vi "Project-1.vi"() -> ()   [LabVIEW 2017]
uses:
  <vilib>/Utility/miscctls.llb/LVPositionTypeDef.ctl
  Control 2.ctl
  System.Speech
panel:
  out "?":bool
  out "?":bool
  out "?":bool
  out "?":bool
  out "Nagasandra":bool
  out "?":bool
  out "?":bool
  out "?":bool
  out "?":bool
  out "Peenya":bool
  out "?":bool
  out "Yeshwantpur":bool
  out "?":bool
  out "Nadaprabhu\nKemepowda, Majestic":bool
  out "National \nCollege":bool
  out "?":bool
  out "?":bool
  out "Jayanagar":bool
  out "?":bool
  out "?":bool
  out "?":bool
  out "?":bool
  out "?":bool
  out "?":bool
  out "Rashtriya Vidyalaya Road":bool
  out "?":bool
  out "Banashankari":bool
  out "?":bool
  out "Jaya Prakash Nagar":bool
  out "TRAIN":bool
  in  "Stop":bool
  out "Yelachenahalli":bool
  # "Yelachenahalli"
  # "Jaya Prakash Nagar"
  # "Banashankari"
  # "Rashtriya Vidyalaya Road"
  # "Jayanagar"
  # "National College"
  # "Nadaprabhu Kempegowda \n     Station, Majestic"
  # "Yeshwantpur"
  # "Peenya"
  # "Nagasandra"
  # "Rashtriya Vidyalaya Road"
  # "Jaya Prakash Nagar"
  # "National College"
  # "Nagasandra"
  # "Yeshwantpur"
  # "Dockyard"
  # "Yelachenahalli"
  # "Nadaprabhu Kempegowda \n     Station, Majestic"
  # "Banashankari"
  # "Jayanagar"
  # "Peenya"
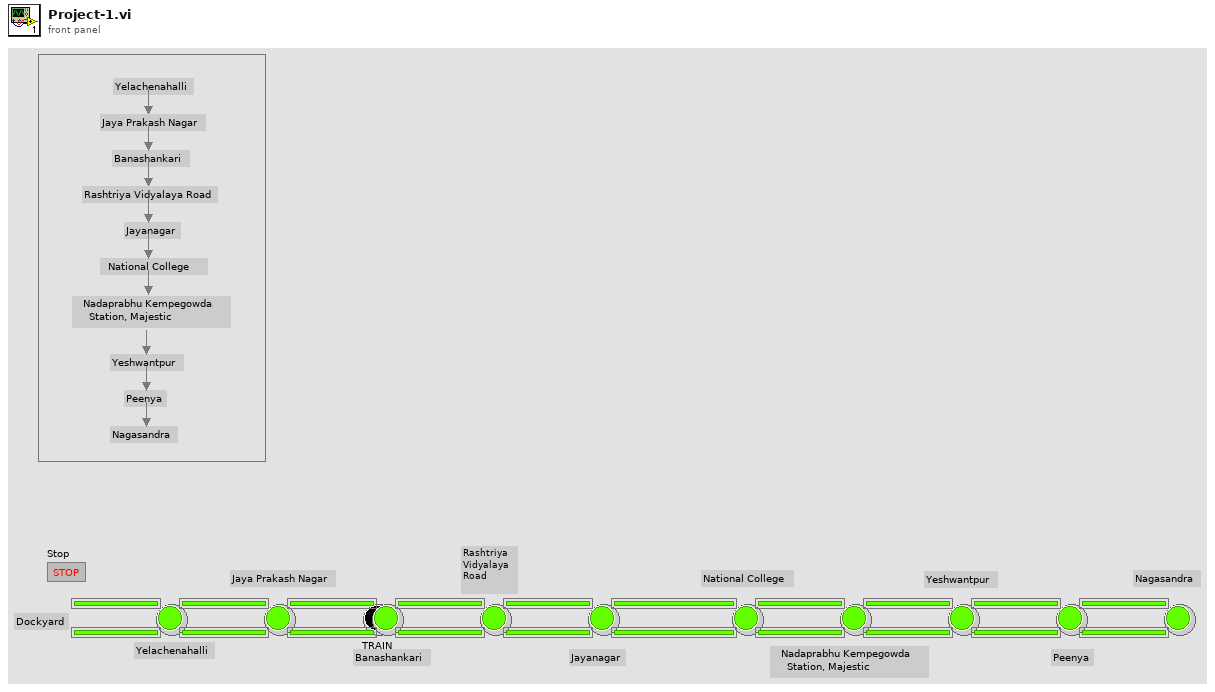
[diagram p1: front panel]
types:
  T1 = typedef "Control 2.ctl" = enum16{"Yelachenahalli", "Jaya Prakash Nagar", "Banashankari", "Rashtriya Vidyalaya Road", "Jayanagar", "National College", "Nadaprabhu Kempegowda Station. Majestic", "Yeshwantpur", "Peenya", "Nagasandra", "Return to Peenya", "Return to Yeshwantpur", "Return to Nadaprabhu Kempegowda Station, Majestic", "Return to National College", "Return to Jayanagar", "Return to Rashtriya Vidyalaya Road", "Return to Banashankari", "Return to Jaya Prakash Nagar", "Return to Yelachenahalli ", "Stop"}
  T2 = typedef "LVPositionTypeDef.ctl" = cluster{"Left":i32, "Top":i32}
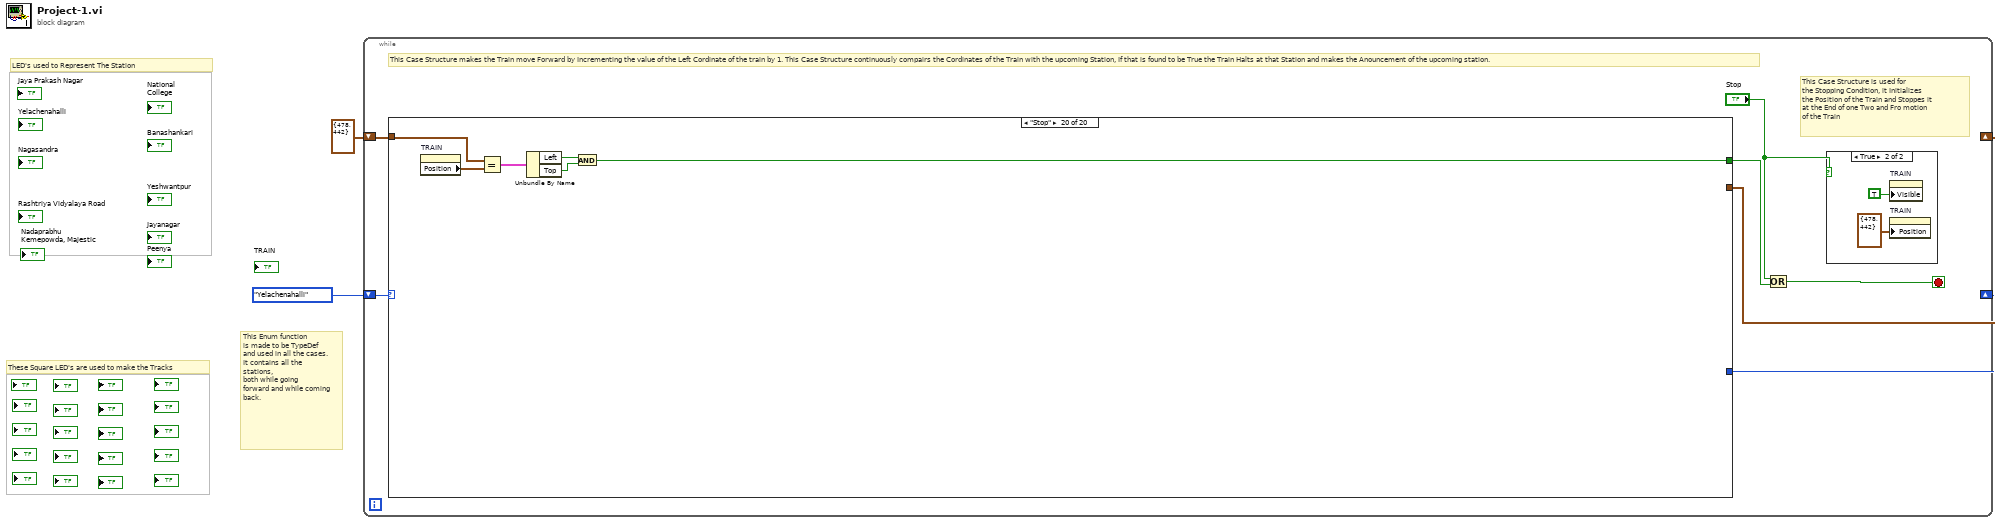
[diagram p0: block diagram]
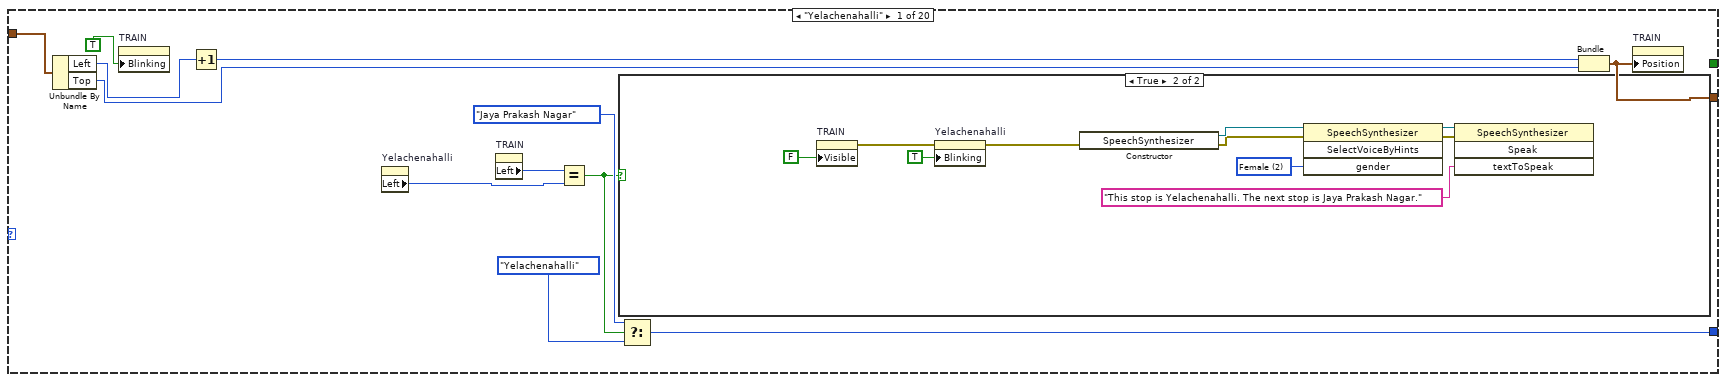
[diagram p2: hidden frame]
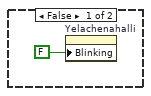
[diagram p3: hidden frame]
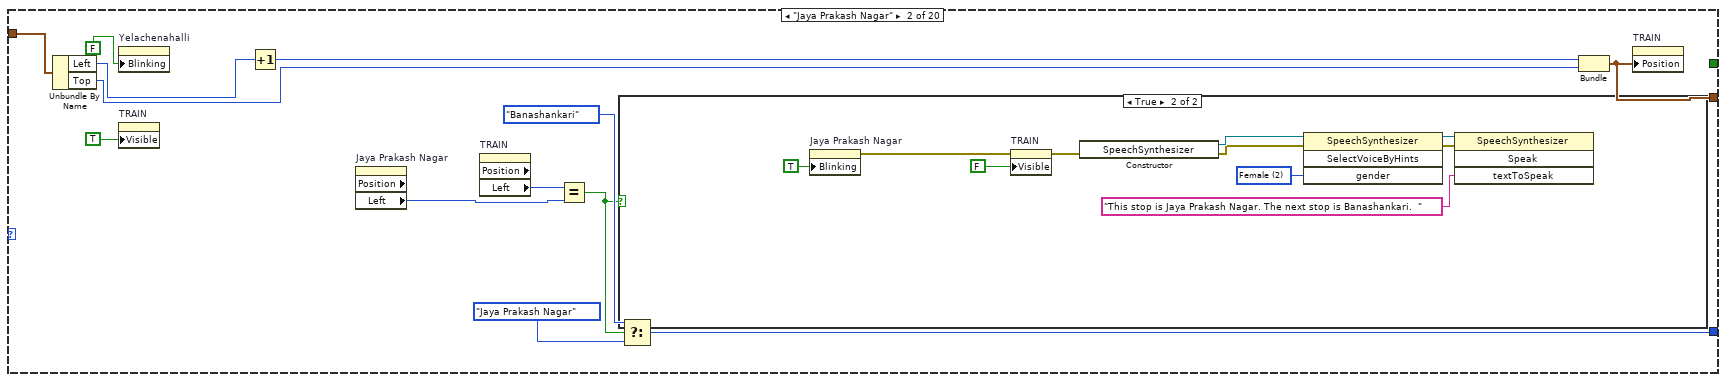
[diagram p4: hidden frame]
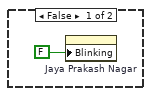
[diagram p5: hidden frame]
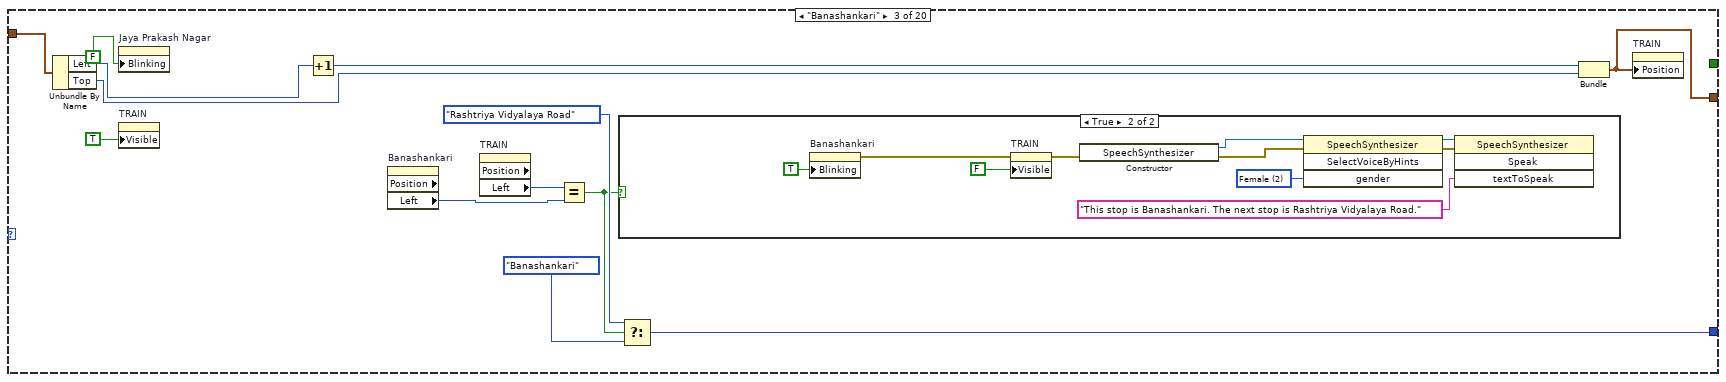
[diagram p6: hidden frame]
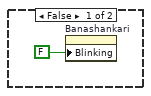
[diagram p7: hidden frame]
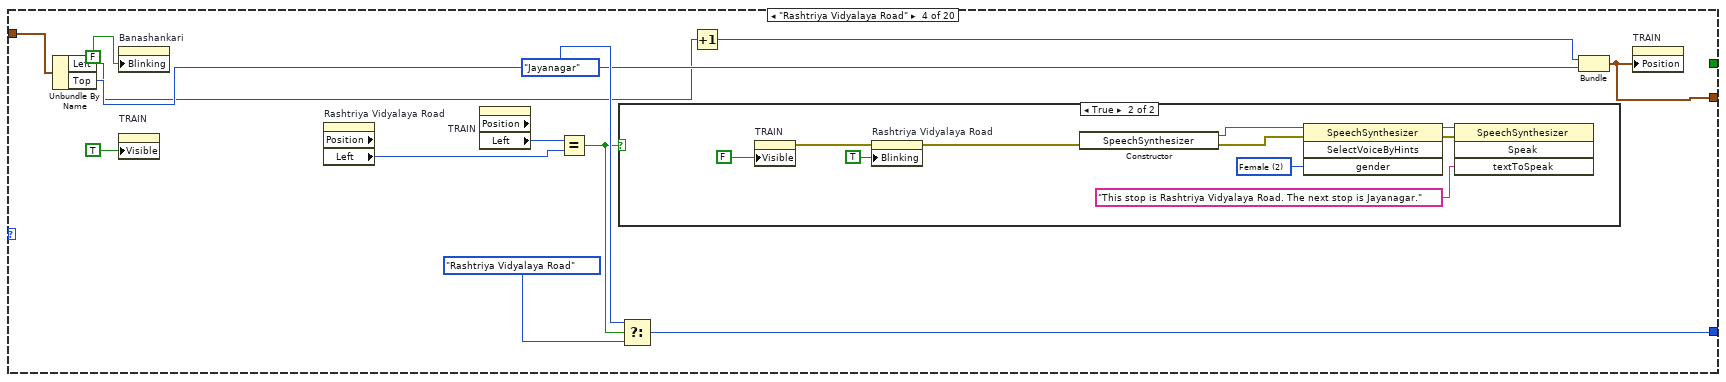
[diagram p8: hidden frame]
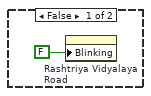
[diagram p9: hidden frame]
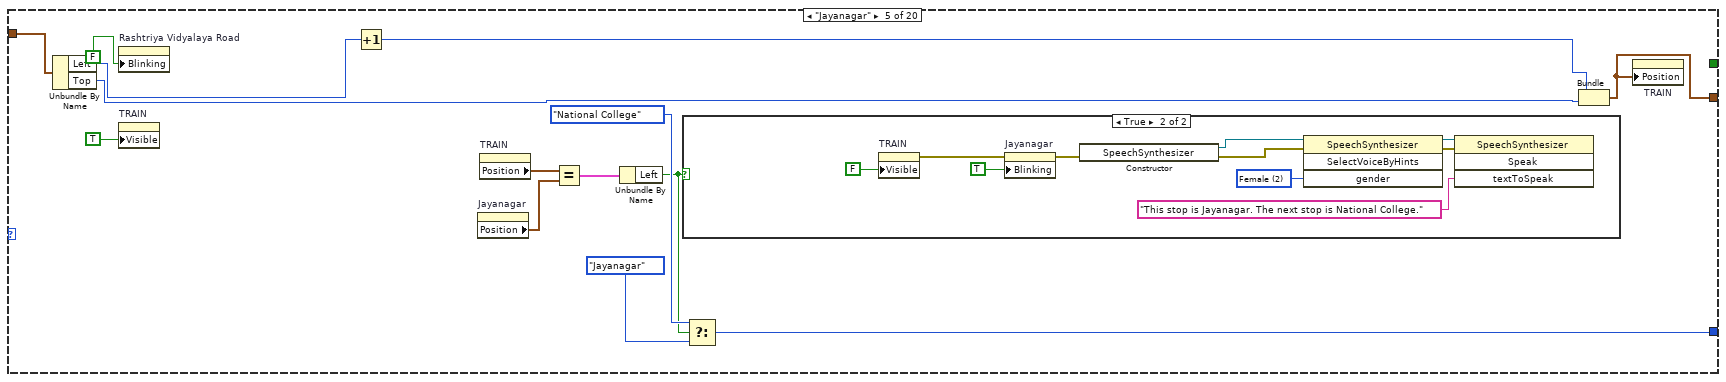
[diagram p10: hidden frame]
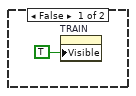
[diagram p11: hidden frame]
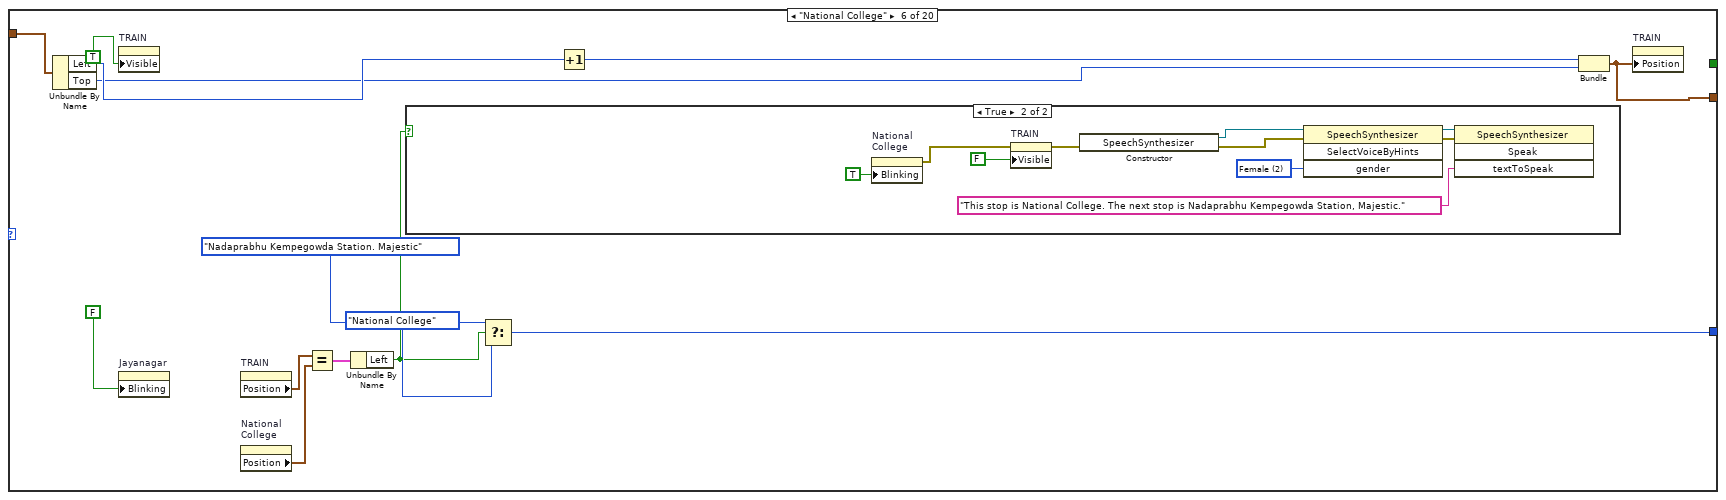
[diagram p12: hidden frame]
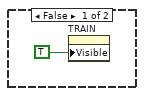
[diagram p13: hidden frame]
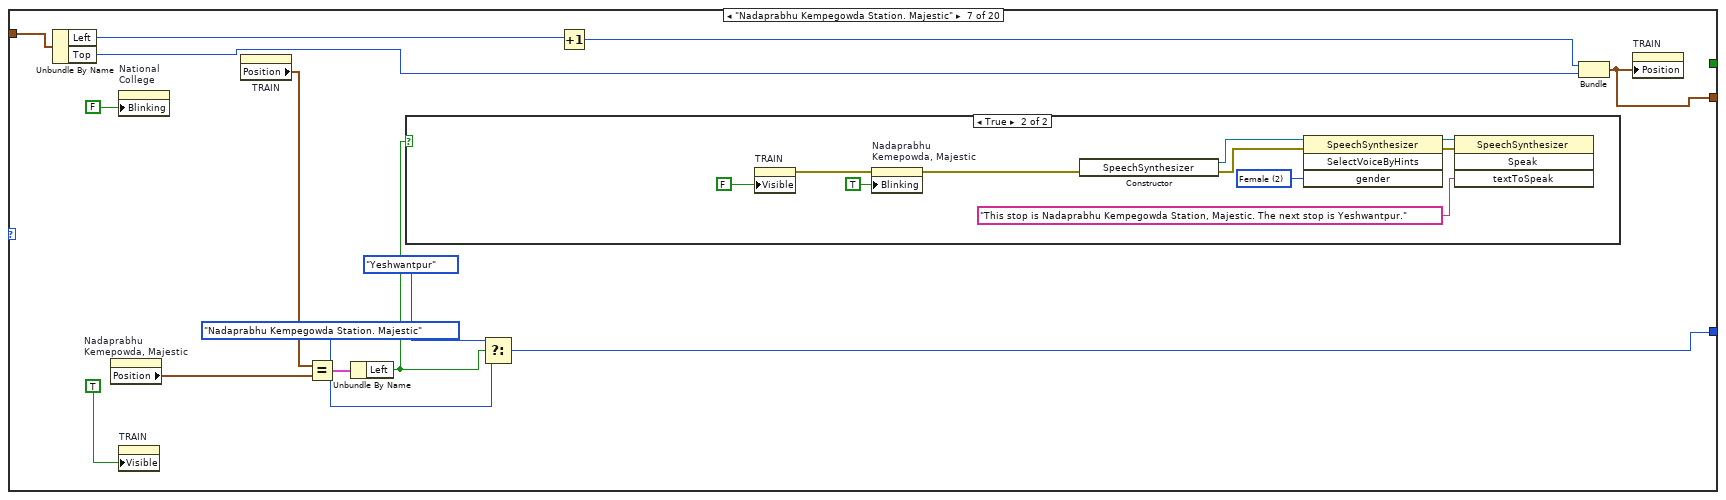
[diagram p14: hidden frame]
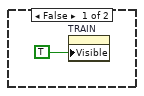
[diagram p15: hidden frame]
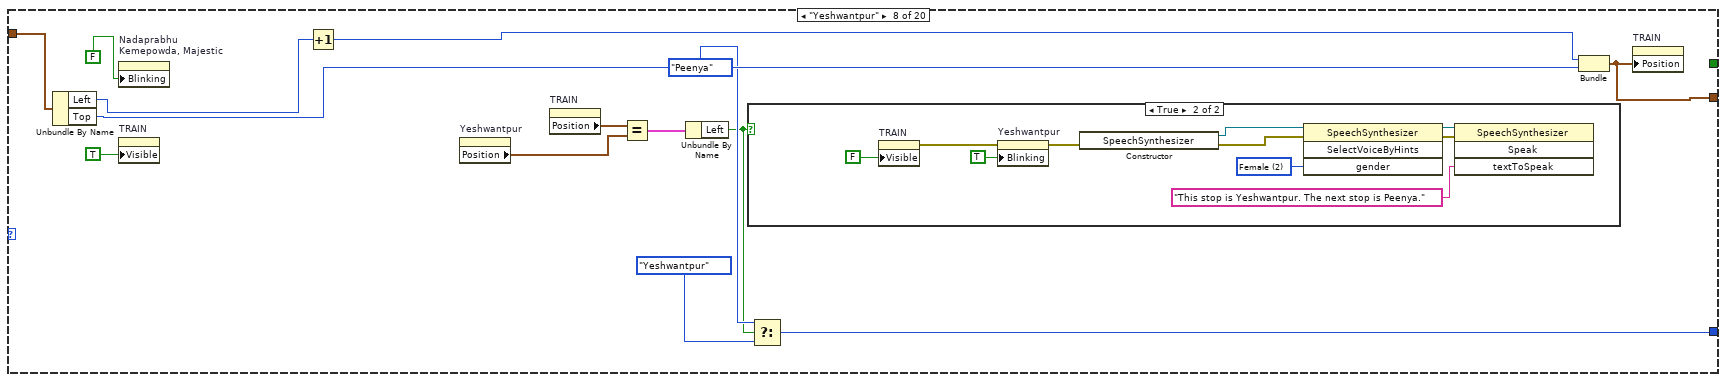
[diagram p16: hidden frame]
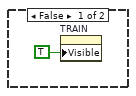
[diagram p17: hidden frame]
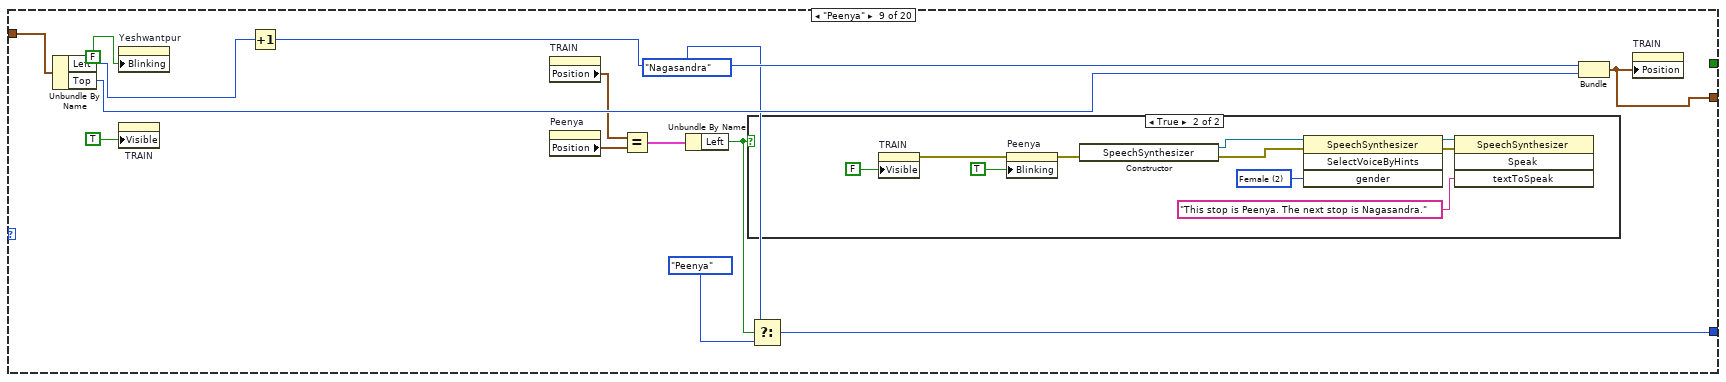
[diagram p18: hidden frame]
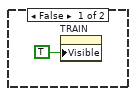
[diagram p19: hidden frame]
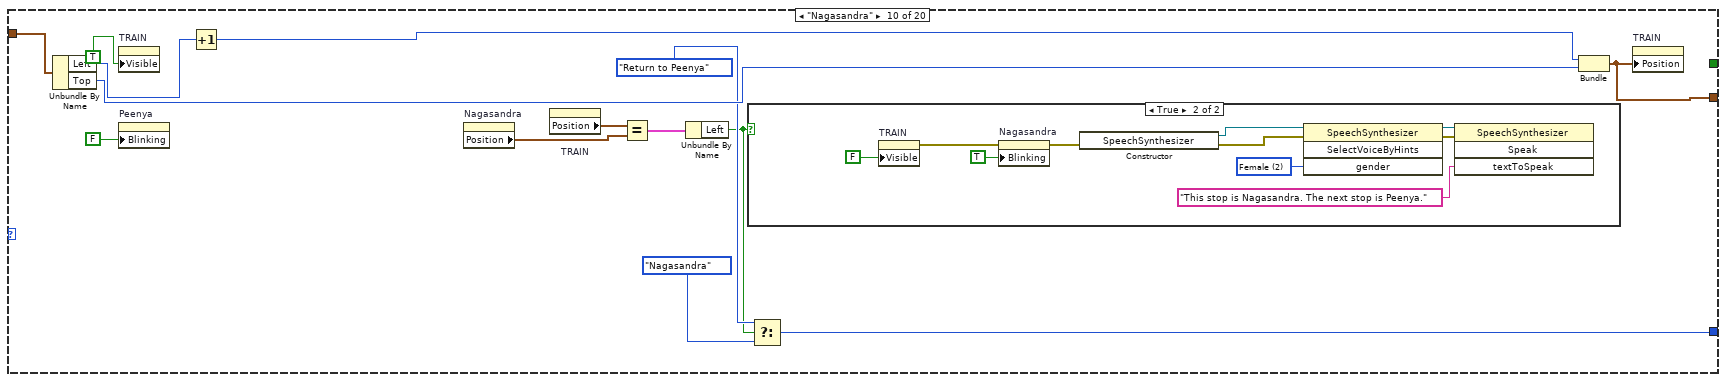
[diagram p20: hidden frame]
diagram:
  # "This Enum function\nis made to be TypeDef\nand used in all the cases.\nIt contains all the stations,\nboth while going\nforward and while coming\nback."
  # "These Square LED's are used to make the Tracks"
  # "LED's used to Represent The Station"
  n1 = while {
    shift-right: [w9] -> _
    shift-left: Control_2."Yelachenahalli" -> [w6]
    shift-right: [w7] -> _
    shift-left: T2 {"Left"=478, "Top"=442} ("Position") -> [w8]
    stop <- w3 stop-if-true
    # "This Case Structure makes the Train move Forward by Incrementing the value of the Left Cordinate of the train by 1. This Case Structure continuously compairs the Cordinates of the Train with the upcoming Station, If that is found to be True the Train Halts at that Station and makes the Anouncement of the upcoming station."
    # "This Case Structure is used for\nthe Stopping Condition, it Initializes\nthe Position of the Train and Stoppes it \nat the End of one Two and Fro motion\nof the Train"
    n2 = case shown="\"Stop\"" w6 {
      tunnel: [w19 w43 w67 w91 w108 w133 w159 w184 w209 w234 w259 w284 w309 w334 w359 w384 w409 w434 w459 _] -> w9
      tunnel: [w11 w33 w57 w81 w112 w137 w162 w187 w212 w237 w262 w287 w312 w337 w362 w387 w412 w437 w462 _] -> w7
      tunnel: w8 -> [w12 w35 w58 w85 w115 w140 w165 w190 w215 w240 w265 w290 w315 w340 w365 w390 w415 w440 w465 w484]
      tunnel: [_ _ _ _ _ _ _ _ _ _ _ _ _ _ _ _ _ _ _ w480] -> w4
      frame "Yelachenahalli" {
        n3 = Unbundle By Name(w12) -> ("Left"=w13:i32, "Top"=w14:i32)
        n4 = property on="TRAIN" class="Bool (strict)"("Blinking"=TRUE) -> ()  [unwired: 2 in, 2 out]
        n5 = Increment(x=w13) -> (x+1=w15:i32)
        n6 = property on="Yelachenahalli" class="Bool (strict)"() -> ("Left"=w17:i32)  [unwired: 2 in, 2 out]
        n7 = property on="TRAIN" class="Bool (strict)"() -> ("Left"=w18:i32)  [unwired: 2 in, 2 out]
        n8 = Equal?(x=w18, y=w17) -> (x = y?=w16:bool)
        n9 = case shown="True" w16 {
          frame False {
            n10 = property on="Yelachenahalli" class="Bool (strict)"("Blinking"=FALSE) -> ()  [unwired: 2 in, 2 out]
          }
          frame True {
            w28 = 2 items=["NotSet", "Male", "Female", "Neutral"] ("gender")
            n11 = property on="TRAIN" class="Bool (strict)"("Visible"=FALSE) -> (error out=w25:errorcluster)  [unwired: 2 in, 1 out]
            n12 = property on="Yelachenahalli" class="Bool (strict)"(error in=w25, "Blinking"=TRUE) -> (error out=w24:errorcluster)  [unwired: 1 in, 1 out]
            n13 = constructor class="SpeechSynthesizer"(error in=w24) -> (reference out=w30:refnum<k24>, error out=w29:errorcluster)  [unwired: 2 in, 1 out]
            n14 = invoke class="SpeechSynthesizer" method="SelectVoiceByHints"(reference=w30, error in=w29, "gender"=w28) -> (reference out=w27:refnum<k24>, error out=w26:errorcluster)  [unwired: 1 in, 2 out]
            n15 = invoke class="SpeechSynthesizer" method="Speak"(reference=w27, error in=w26, "textToSpeak"="This stop is Yelachenahalli. The next stop is Jaya Prakash Nagar.") -> ()  [unwired: 1 in, 4 out]
          }
        }
        n16 = Select(t=Control_2."Jaya Prakash Nagar", s=w16, f=Control_2."Yelachenahalli") -> (s? t:f=w19:T1)
        n17 = Bundle(w15, "Top"=w14) -> (w11:cluster{i32, "Top":i32})  [unwired: 1 in]
        n18 = property on="TRAIN" class="Bool (strict)"("Position"=w11) -> ()  [unwired: 2 in, 2 out]
      }
      frame "Jaya Prakash Nagar" {
        n19 = Unbundle By Name(w35) -> ("Left"=w34:i32, "Top"=w36:i32)
        n20 = property on="Yelachenahalli" class="Bool (strict)"("Blinking"=FALSE) -> ()  [unwired: 2 in, 2 out]
        n21 = property on="TRAIN" class="Bool (strict)"("Visible"=TRUE) -> ()  [unwired: 2 in, 2 out]
        n22 = Increment(x=w34) -> (x+1=w37:i32)
        n23 = property on="Jaya Prakash Nagar" class="Bool (strict)" props=["Position", "Left"]() -> ("Left"=w41:i32)  [unwired: 2 in, 3 out]
        n24 = property on="TRAIN" class="Bool (strict)" props=["Position", "Left"]() -> ("Left"=w42:i32)  [unwired: 2 in, 3 out]
        n25 = Equal?(x=w42, y=w41) -> (x = y?=w40:bool)
        n26 = case shown="True" w40 {
          frame False {
            n27 = property on="Jaya Prakash Nagar" class="Bool (strict)"("Blinking"=FALSE) -> ()  [unwired: 2 in, 2 out]
          }
          frame True {
            w53 = 2 items=["NotSet", "Male", "Female", "Neutral"] ("gender")
            n28 = property on="Jaya Prakash Nagar" class="Bool (strict)"("Blinking"=TRUE) -> (error out=w48:errorcluster)  [unwired: 2 in, 1 out]
            n29 = property on="TRAIN" class="Bool (strict)"(error in=w48, "Visible"=FALSE) -> (error out=w49:errorcluster)  [unwired: 1 in, 1 out]
            n30 = constructor class="SpeechSynthesizer"(error in=w49) -> (reference out=w55:refnum<k24>, error out=w54:errorcluster)  [unwired: 2 in, 1 out]
            n31 = invoke class="SpeechSynthesizer" method="SelectVoiceByHints"(reference=w55, error in=w54, "gender"=w53) -> (reference out=w52:refnum<k24>, error out=w51:errorcluster)  [unwired: 1 in, 2 out]
            n32 = invoke class="SpeechSynthesizer" method="Speak"(reference=w52, error in=w51, "textToSpeak"="This stop is Jaya Prakash Nagar. The next stop is Banashankari.  ") -> ()  [unwired: 1 in, 4 out]
          }
        }
        n33 = Select(t=Control_2."Banashankari", s=w40, f=Control_2."Jaya Prakash Nagar") -> (s? t:f=w43:T1)
        n34 = Bundle(w37, "Top"=w36) -> (w33:cluster{i32, "Top":i32})  [unwired: 1 in]
        n35 = property on="TRAIN" class="Bool (strict)"("Position"=w33) -> ()  [unwired: 2 in, 2 out]
      }
      frame "Banashankari" {
        n36 = Unbundle By Name(w58) -> ("Left"=w59:i32, "Top"=w60:i32)
        n37 = property on="Jaya Prakash Nagar" class="Bool (strict)"("Blinking"=FALSE) -> ()  [unwired: 2 in, 2 out]
        n38 = property on="TRAIN" class="Bool (strict)"("Visible"=TRUE) -> ()  [unwired: 2 in, 2 out]
        n39 = Increment(x=w59) -> (x+1=w61:i32)
        n40 = property on="Banashankari" class="Bool (strict)" props=["Position", "Left"]() -> ("Left"=w65:i32)  [unwired: 2 in, 3 out]
        n41 = property on="TRAIN" class="Bool (strict)" props=["Position", "Left"]() -> ("Left"=w66:i32)  [unwired: 2 in, 3 out]
        n42 = Equal?(x=w66, y=w65) -> (x = y?=w64:bool)
        n43 = case shown="True" w64 {
          frame False {
            n44 = property on="Banashankari" class="Bool (strict)"("Blinking"=FALSE) -> ()  [unwired: 2 in, 2 out]
          }
          frame True {
            w77 = 2 items=["NotSet", "Male", "Female", "Neutral"] ("gender")
            n45 = property on="Banashankari" class="Bool (strict)"("Blinking"=TRUE) -> (error out=w71:errorcluster)  [unwired: 2 in, 1 out]
            n46 = property on="TRAIN" class="Bool (strict)"(error in=w71, "Visible"=FALSE) -> (error out=w72:errorcluster)  [unwired: 1 in, 1 out]
            n47 = constructor class="SpeechSynthesizer"(error in=w72) -> (reference out=w75:refnum<k24>, error out=w76:errorcluster)  [unwired: 2 in, 1 out]
            n48 = invoke class="SpeechSynthesizer" method="SelectVoiceByHints"(reference=w75, error in=w76, "gender"=w77) -> (reference out=w73:refnum<k24>, error out=w78:errorcluster)  [unwired: 1 in, 2 out]
            n49 = invoke class="SpeechSynthesizer" method="Speak"(reference=w73, error in=w78, "textToSpeak"="This stop is Banashankari. The next stop is Rashtriya Vidyalaya Road.") -> ()  [unwired: 1 in, 4 out]
          }
        }
        n50 = Select(t=Control_2."Rashtriya Vidyalaya Road", s=w64, f=Control_2."Banashankari") -> (s? t:f=w67:T1)
        n51 = Bundle(w61, "Top"=w60) -> (w57:cluster{i32, "Top":i32})  [unwired: 1 in]
        n52 = property on="TRAIN" class="Bool (strict)"("Position"=w57) -> ()  [unwired: 2 in, 2 out]
      }
      frame "Rashtriya Vidyalaya Road" {
        n53 = Unbundle By Name(w85) -> ("Left"=w82:i32, "Top"=w83:i32)
        n54 = property on="Banashankari" class="Bool (strict)"("Blinking"=FALSE) -> ()  [unwired: 2 in, 2 out]
        n55 = property on="TRAIN" class="Bool (strict)"("Visible"=TRUE) -> ()  [unwired: 2 in, 2 out]
        n56 = property on="Rashtriya Vidyalaya Road" class="Bool (strict)" props=["Position", "Left"]() -> ("Left"=w89:i32)  [unwired: 2 in, 3 out]
        n57 = property on="TRAIN" class="Bool (strict)" props=["Position", "Left"]() -> ("Left"=w90:i32)  [unwired: 2 in, 3 out]
        n58 = Equal?(x=w90, y=w89) -> (x = y?=w88:bool)
        n59 = case shown="True" w88 {
          frame False {
            n60 = property on="Rashtriya Vidyalaya Road" class="Bool (strict)"("Blinking"=FALSE) -> ()  [unwired: 2 in, 2 out]
          }
          frame True {
            w101 = 2 items=["NotSet", "Male", "Female", "Neutral"] ("gender")
            n61 = property on="TRAIN" class="Bool (strict)"("Visible"=FALSE) -> (error out=w95:errorcluster)  [unwired: 2 in, 1 out]
            n62 = property on="Rashtriya Vidyalaya Road" class="Bool (strict)"(error in=w95, "Blinking"=TRUE) -> (error out=w96:errorcluster)  [unwired: 1 in, 1 out]
            n63 = constructor class="SpeechSynthesizer"(error in=w96) -> (reference out=w99:refnum<k24>, error out=w100:errorcluster)  [unwired: 2 in, 1 out]
            n64 = invoke class="SpeechSynthesizer" method="SelectVoiceByHints"(reference=w99, error in=w100, "gender"=w101) -> (reference out=w98:refnum<k24>, error out=w102:errorcluster)  [unwired: 1 in, 2 out]
            n65 = invoke class="SpeechSynthesizer" method="Speak"(reference=w98, error in=w102, "textToSpeak"="This stop is Rashtriya Vidyalaya Road. The next stop is Jayanagar.") -> ()  [unwired: 1 in, 4 out]
          }
        }
        n66 = Select(t=Control_2."Jayanagar", s=w88, f=Control_2."Rashtriya Vidyalaya Road") -> (s? t:f=w91:T1)
        n67 = Increment(x=w82) -> (x+1=w84:i32)
        n68 = Bundle(w84, "Top"=w83) -> (w81:cluster{i32, "Top":i32})  [unwired: 1 in]
        n69 = property on="TRAIN" class="Bool (strict)"("Position"=w81) -> ()  [unwired: 2 in, 2 out]
      }
      frame "Jayanagar" {
        n70 = Unbundle By Name(w115) -> ("Left"=w118:i32, "Top"=w117:i32)
        n71 = property on="Rashtriya Vidyalaya Road" class="Bool (strict)"("Blinking"=FALSE) -> ()  [unwired: 2 in, 2 out]
        n72 = property on="TRAIN" class="Bool (strict)"("Visible"=TRUE) -> ()  [unwired: 2 in, 2 out]
        n73 = Increment(x=w118) -> (x+1=w116:i32)
        n74 = property on="Jayanagar" class="Bool (strict)"() -> ("Position"=w105:T2)  [unwired: 2 in, 2 out]
        n75 = property on="TRAIN" class="Bool (strict)"() -> ("Position"=w110:T2)  [unwired: 2 in, 2 out]
        n76 = Equal?(x=w110, y=w105) -> (x = y?=w111:cluster{"Left":bool, "Top":bool})
        n77 = Unbundle By Name(w111) -> ("Left"=w107:bool)
        n78 = case shown="True" w107 {
          frame False {
            n79 = property on="TRAIN" class="Bool (strict)"("Visible"=TRUE) -> ()  [unwired: 2 in, 2 out]
          }
          frame True {
            w126 = 2 items=["NotSet", "Male", "Female", "Neutral"] ("gender")
            n80 = property on="TRAIN" class="Bool (strict)"("Visible"=FALSE) -> (error out=w120:errorcluster)  [unwired: 2 in, 1 out]
            n81 = property on="Jayanagar" class="Bool (strict)"(error in=w120, "Blinking"=TRUE) -> (error out=w121:errorcluster)  [unwired: 1 in, 1 out]
            n82 = constructor class="SpeechSynthesizer"(error in=w121) -> (reference out=w124:refnum<k24>, error out=w125:errorcluster)  [unwired: 2 in, 1 out]
            n83 = invoke class="SpeechSynthesizer" method="SelectVoiceByHints"(reference=w124, error in=w125, "gender"=w126) -> (reference out=w123:refnum<k24>, error out=w127:errorcluster)  [unwired: 1 in, 2 out]
            n84 = invoke class="SpeechSynthesizer" method="Speak"(reference=w123, error in=w127, "textToSpeak"="This stop is Jayanagar. The next stop is National College.") -> ()  [unwired: 1 in, 4 out]
          }
        }
        n85 = Select(t=Control_2."National College", s=w107, f=Control_2."Jayanagar") -> (s? t:f=w108:T1)
        n86 = Bundle(w116, "Top"=w117) -> (w112:cluster{i32, "Top":i32})  [unwired: 1 in]
        n87 = property on="TRAIN" class="Bool (strict)"("Position"=w112) -> ()  [unwired: 2 in, 2 out]
      }
      frame "National College" {
        n88 = Unbundle By Name(w140) -> ("Left"=w143:i32, "Top"=w142:i32)
        n89 = property on="TRAIN" class="Bool (strict)"("Visible"=TRUE) -> ()  [unwired: 2 in, 2 out]
        n90 = property on="Jayanagar" class="Bool (strict)"("Blinking"=FALSE) -> ()  [unwired: 2 in, 2 out]
        n91 = property on="TRAIN" class="Bool (strict)"() -> ("Position"=w135:T2)  [unwired: 2 in, 2 out]
        n92 = property on="National \nCollege" class="Bool (strict)"() -> ("Position"=w130:T2)  [unwired: 2 in, 2 out]
        n93 = Equal?(x=w135, y=w130) -> (x = y?=w136:cluster{"Left":bool, "Top":bool})
        n94 = Unbundle By Name(w136) -> ("Left"=w132:bool)
        n95 = case shown="True" w132 {
          frame False {
            n96 = property on="TRAIN" class="Bool (strict)"("Visible"=TRUE) -> ()  [unwired: 2 in, 2 out]
          }
          frame True {
            w151 = 2 items=["NotSet", "Male", "Female", "Neutral"] ("gender")
            n97 = property on="National \nCollege" class="Bool (strict)"("Blinking"=TRUE) -> (error out=w145:errorcluster)  [unwired: 2 in, 1 out]
            n98 = property on="TRAIN" class="Bool (strict)"(error in=w145, "Visible"=FALSE) -> (error out=w146:errorcluster)  [unwired: 1 in, 1 out]
            n99 = constructor class="SpeechSynthesizer"(error in=w146) -> (reference out=w149:refnum<k24>, error out=w150:errorcluster)  [unwired: 2 in, 1 out]
            n100 = invoke class="SpeechSynthesizer" method="SelectVoiceByHints"(reference=w149, error in=w150, "gender"=w151) -> (reference out=w147:refnum<k24>, error out=w152:errorcluster)  [unwired: 1 in, 2 out]
            n101 = invoke class="SpeechSynthesizer" method="Speak"(reference=w147, error in=w152, "textToSpeak"="This stop is National College. The next stop is Nadaprabhu Kempegowda Station, Majestic.") -> ()  [unwired: 1 in, 4 out]
          }
        }
        n102 = Select(t=Control_2."Nadaprabhu Kempegowda Station. Majestic", s=w132, f=Control_2."National College") -> (s? t:f=w133:T1)
        n103 = Increment(x=w143) -> (x+1=w141:i32)
        n104 = Bundle(w141, "Top"=w142) -> (w137:cluster{i32, "Top":i32})  [unwired: 1 in]
        n105 = property on="TRAIN" class="Bool (strict)"("Position"=w137) -> ()  [unwired: 2 in, 2 out]
      }
      frame "Nadaprabhu Kempegowda Station. Majestic" {
        n106 = Unbundle By Name(w165) -> ("Left"=w168:i32, "Top"=w167:i32)
        n107 = property on="Nadaprabhu\nKemepowda, Majestic" class="Bool (strict)"() -> ("Position"=w155:T2)  [unwired: 2 in, 2 out]
        n108 = property on="National \nCollege" class="Bool (strict)"("Blinking"=FALSE) -> ()  [unwired: 2 in, 2 out]
        n109 = property on="TRAIN" class="Bool (strict)"("Visible"=TRUE) -> ()  [unwired: 2 in, 2 out]
        n110 = property on="TRAIN" class="Bool (strict)"() -> ("Position"=w160:T2)  [unwired: 2 in, 2 out]
        n111 = Equal?(x=w160, y=w155) -> (x = y?=w161:cluster{"Left":bool, "Top":bool})
        n112 = Unbundle By Name(w161) -> ("Left"=w158:bool)
        n113 = case shown="True" w158 {
          frame False {
            n114 = property on="TRAIN" class="Bool (strict)"("Visible"=TRUE) -> ()  [unwired: 2 in, 2 out]
          }
          frame True {
            w176 = 2 items=["NotSet", "Male", "Female", "Neutral"] ("gender")
            n115 = property on="TRAIN" class="Bool (strict)"("Visible"=FALSE) -> (error out=w170:errorcluster)  [unwired: 2 in, 1 out]
            n116 = property on="Nadaprabhu\nKemepowda, Majestic" class="Bool (strict)"(error in=w170, "Blinking"=TRUE) -> (error out=w171:errorcluster)  [unwired: 1 in, 1 out]
            n117 = constructor class="SpeechSynthesizer"(error in=w171) -> (reference out=w174:refnum<k24>, error out=w175:errorcluster)  [unwired: 2 in, 1 out]
            n118 = invoke class="SpeechSynthesizer" method="SelectVoiceByHints"(reference=w174, error in=w175, "gender"=w176) -> (reference out=w172:refnum<k24>, error out=w177:errorcluster)  [unwired: 1 in, 2 out]
            n119 = invoke class="SpeechSynthesizer" method="Speak"(reference=w172, error in=w177, "textToSpeak"="This stop is Nadaprabhu Kempegowda Station, Majestic. The next stop is Yeshwantpur.") -> ()  [unwired: 1 in, 4 out]
          }
        }
        n120 = Select(t=Control_2."Yeshwantpur", s=w158, f=Control_2."Nadaprabhu Kempegowda Station. Majestic") -> (s? t:f=w159:T1)
        n121 = Increment(x=w168) -> (x+1=w166:i32)
        n122 = Bundle(w166, "Top"=w167) -> (w162:cluster{i32, "Top":i32})  [unwired: 1 in]
        n123 = property on="TRAIN" class="Bool (strict)"("Position"=w162) -> ()  [unwired: 2 in, 2 out]
      }
      frame "Yeshwantpur" {
        n124 = Unbundle By Name(w190) -> ("Left"=w193:i32, "Top"=w192:i32)
        n125 = property on="Nadaprabhu\nKemepowda, Majestic" class="Bool (strict)"("Blinking"=FALSE) -> ()  [unwired: 2 in, 2 out]
        n126 = property on="TRAIN" class="Bool (strict)"("Visible"=TRUE) -> ()  [unwired: 2 in, 2 out]
        n127 = Increment(x=w193) -> (x+1=w191:i32)
        n128 = property on="Yeshwantpur" class="Bool (strict)"() -> ("Position"=w180:T2)  [unwired: 2 in, 2 out]
        n129 = property on="TRAIN" class="Bool (strict)"() -> ("Position"=w185:T2)  [unwired: 2 in, 2 out]
        n130 = Equal?(x=w185, y=w180) -> (x = y?=w186:cluster{"Left":bool, "Top":bool})
        n131 = Unbundle By Name(w186) -> ("Left"=w183:bool)
        n132 = case shown="True" w183 {
          frame False {
            n133 = property on="TRAIN" class="Bool (strict)"("Visible"=TRUE) -> ()  [unwired: 2 in, 2 out]
          }
          frame True {
            w201 = 2 items=["NotSet", "Male", "Female", "Neutral"] ("gender")
            n134 = property on="TRAIN" class="Bool (strict)"("Visible"=FALSE) -> (error out=w195:errorcluster)  [unwired: 2 in, 1 out]
            n135 = property on="Yeshwantpur" class="Bool (strict)"(error in=w195, "Blinking"=TRUE) -> (error out=w196:errorcluster)  [unwired: 1 in, 1 out]
            n136 = constructor class="SpeechSynthesizer"(error in=w196) -> (reference out=w199:refnum<k24>, error out=w200:errorcluster)  [unwired: 2 in, 1 out]
            n137 = invoke class="SpeechSynthesizer" method="SelectVoiceByHints"(reference=w199, error in=w200, "gender"=w201) -> (reference out=w198:refnum<k24>, error out=w202:errorcluster)  [unwired: 1 in, 2 out]
            n138 = invoke class="SpeechSynthesizer" method="Speak"(reference=w198, error in=w202, "textToSpeak"="This stop is Yeshwantpur. The next stop is Peenya.") -> ()  [unwired: 1 in, 4 out]
          }
        }
        n139 = Select(t=Control_2."Peenya", s=w183, f=Control_2."Yeshwantpur") -> (s? t:f=w184:T1)
        n140 = Bundle(w191, "Top"=w192) -> (w187:cluster{i32, "Top":i32})  [unwired: 1 in]
        n141 = property on="TRAIN" class="Bool (strict)"("Position"=w187) -> ()  [unwired: 2 in, 2 out]
      }
      frame "Peenya" {
        n142 = Unbundle By Name(w215) -> ("Left"=w218:i32, "Top"=w217:i32)
        n143 = property on="Yeshwantpur" class="Bool (strict)"("Blinking"=FALSE) -> ()  [unwired: 2 in, 2 out]
        n144 = property on="TRAIN" class="Bool (strict)"("Visible"=TRUE) -> ()  [unwired: 2 in, 2 out]
        n145 = Increment(x=w218) -> (x+1=w216:i32)
        n146 = property on="TRAIN" class="Bool (strict)"() -> ("Position"=w210:T2)  [unwired: 2 in, 2 out]
        n147 = property on="Peenya" class="Bool (strict)"() -> ("Position"=w205:T2)  [unwired: 2 in, 2 out]
        n148 = Equal?(x=w210, y=w205) -> (x = y?=w211:cluster{"Left":bool, "Top":bool})
        n149 = Unbundle By Name(w211) -> ("Left"=w208:bool)
        n150 = case shown="True" w208 {
          frame False {
            n151 = property on="TRAIN" class="Bool (strict)"("Visible"=TRUE) -> ()  [unwired: 2 in, 2 out]
          }
          frame True {
            w226 = 2 items=["NotSet", "Male", "Female", "Neutral"] ("gender")
            n152 = property on="TRAIN" class="Bool (strict)"("Visible"=FALSE) -> (error out=w220:errorcluster)  [unwired: 2 in, 1 out]
            n153 = property on="Peenya" class="Bool (strict)"(error in=w220, "Blinking"=TRUE) -> (error out=w221:errorcluster)  [unwired: 1 in, 1 out]
            n154 = constructor class="SpeechSynthesizer"(error in=w221) -> (reference out=w224:refnum<k24>, error out=w225:errorcluster)  [unwired: 2 in, 1 out]
            n155 = invoke class="SpeechSynthesizer" method="SelectVoiceByHints"(reference=w224, error in=w225, "gender"=w226) -> (reference out=w223:refnum<k24>, error out=w227:errorcluster)  [unwired: 1 in, 2 out]
            n156 = invoke class="SpeechSynthesizer" method="Speak"(reference=w223, error in=w227, "textToSpeak"="This stop is Peenya. The next stop is Nagasandra.") -> ()  [unwired: 1 in, 4 out]
          }
        }
        n157 = Select(t=Control_2."Nagasandra", s=w208, f=Control_2."Peenya") -> (s? t:f=w209:T1)
        n158 = Bundle(w216, "Top"=w217) -> (w212:cluster{i32, "Top":i32})  [unwired: 1 in]
        n159 = property on="TRAIN" class="Bool (strict)"("Position"=w212) -> ()  [unwired: 2 in, 2 out]
      }
      frame "Nagasandra" {
        n160 = Unbundle By Name(w240) -> ("Left"=w243:i32, "Top"=w242:i32)
        n161 = property on="TRAIN" class="Bool (strict)"("Visible"=TRUE) -> ()  [unwired: 2 in, 2 out]
        n162 = property on="Peenya" class="Bool (strict)"("Blinking"=FALSE) -> ()  [unwired: 2 in, 2 out]
        n163 = Increment(x=w243) -> (x+1=w241:i32)
        n164 = property on="Nagasandra" class="Bool (strict)"() -> ("Position"=w230:T2)  [unwired: 2 in, 2 out]
        n165 = property on="TRAIN" class="Bool (strict)"() -> ("Position"=w235:T2)  [unwired: 2 in, 2 out]
        n166 = Equal?(x=w235, y=w230) -> (x = y?=w236:cluster{"Left":bool, "Top":bool})
        n167 = Unbundle By Name(w236) -> ("Left"=w233:bool)
        n168 = case shown="True" w233 {
          frame False {
            n169 = property on="TRAIN" class="Bool (strict)"("Visible"=TRUE) -> ()  [unwired: 2 in, 2 out]
          }
          frame True {
            w252 = 2 items=["NotSet", "Male", "Female", "Neutral"] ("gender")
            n170 = property on="TRAIN" class="Bool (strict)"("Visible"=FALSE) -> (error out=w245:errorcluster)  [unwired: 2 in, 1 out]
            n171 = property on="Nagasandra" class="Bool (strict)"(error in=w245, "Blinking"=TRUE) -> (error out=w246:errorcluster)  [unwired: 1 in, 1 out]
            n172 = constructor class="SpeechSynthesizer"(error in=w246) -> (reference out=w250:refnum<k24>, error out=w251:errorcluster)  [unwired: 2 in, 1 out]
            n173 = invoke class="SpeechSynthesizer" method="SelectVoiceByHints"(reference=w250, error in=w251, "gender"=w252) -> (reference out=w249:refnum<k24>, error out=w253:errorcluster)  [unwired: 1 in, 2 out]
            n174 = invoke class="SpeechSynthesizer" method="Speak"(reference=w249, error in=w253, "textToSpeak"="This stop is Nagasandra. The next stop is Peenya.") -> ()  [unwired: 1 in, 4 out]
          }
        }
        n175 = Select(t=Control_2."Return to Peenya", s=w233, f=Control_2."Nagasandra") -> (s? t:f=w234:T1)
        n176 = Bundle(w241, "Top"=w242) -> (w237:cluster{i32, "Top":i32})  [unwired: 1 in]
        n177 = property on="TRAIN" class="Bool (strict)"("Position"=w237) -> ()  [unwired: 2 in, 2 out]
      }
      frame "Return to Peenya" {
        n178 = Unbundle By Name(w265) -> ("Left"=w268:i32, "Top"=w267:i32)
        n179 = property on="Nagasandra" class="Bool (strict)"("Blinking"=FALSE) -> ()  [unwired: 2 in, 2 out]
        n180 = property on="TRAIN" class="Bool (strict)"("Visible"=TRUE) -> ()  [unwired: 2 in, 2 out]
        n181 = Decrement(x=w268) -> (x-1=w266:i32)
        n182 = property on="TRAIN" class="Bool (strict)"() -> ("Position"=w260:T2)  [unwired: 2 in, 2 out]
        n183 = property on="Peenya" class="Bool (strict)"() -> ("Position"=w255:T2)  [unwired: 2 in, 2 out]
        n184 = Equal?(x=w260, y=w255) -> (x = y?=w261:cluster{"Left":bool, "Top":bool})
        n185 = Unbundle By Name(w261) -> ("Left"=w258:bool)
        n186 = case shown="True" w258 {
          frame False {
            n187 = property on="TRAIN" class="Bool (strict)"("Visible"=TRUE) -> ()  [unwired: 2 in, 2 out]
          }
          frame True {
            w276 = 2 items=["NotSet", "Male", "Female", "Neutral"] ("gender")
            n188 = property on="TRAIN" class="Bool (strict)"("Visible"=FALSE) -> (error out=w270:errorcluster)  [unwired: 2 in, 1 out]
            n189 = property on="Peenya" class="Bool (strict)"(error in=w270, "Blinking"=TRUE) -> (error out=w271:errorcluster)  [unwired: 1 in, 1 out]
            n190 = constructor class="SpeechSynthesizer"(error in=w271) -> (reference out=w274:refnum<k24>, error out=w275:errorcluster)  [unwired: 2 in, 1 out]
            n191 = invoke class="SpeechSynthesizer" method="SelectVoiceByHints"(reference=w274, error in=w275, "gender"=w276) -> (reference out=w273:refnum<k24>, error out=w277:errorcluster)  [unwired: 1 in, 2 out]
            n192 = invoke class="SpeechSynthesizer" method="Speak"(reference=w273, error in=w277, "textToSpeak"="This stop is Peenya. The next stop is Yeshwantpur.") -> ()  [unwired: 1 in, 4 out]
          }
        }
        n193 = Select(t=Control_2."Return to Yeshwantpur", s=w258, f=Control_2."Return to Peenya") -> (s? t:f=w259:T1)
        n194 = Bundle(w266, "Top"=w267) -> (w262:cluster{i32, "Top":i32})  [unwired: 1 in]
        n195 = property on="TRAIN" class="Bool (strict)"("Position"=w262) -> ()  [unwired: 2 in, 2 out]
      }
      frame "Return to Yeshwantpur" {
        n196 = Unbundle By Name(w290) -> ("Left"=w293:i32, "Top"=w292:i32)
        n197 = property on="TRAIN" class="Bool (strict)"("Visible"=TRUE) -> ()  [unwired: 2 in, 2 out]
        n198 = property on="Peenya" class="Bool (strict)"("Blinking"=FALSE) -> ()  [unwired: 2 in, 2 out]
        n199 = property on="Yeshwantpur" class="Bool (strict)"() -> ("Position"=w280:T2)  [unwired: 2 in, 2 out]
        n200 = property on="TRAIN" class="Bool (strict)"() -> ("Position"=w285:T2)  [unwired: 2 in, 2 out]
        n201 = Equal?(x=w285, y=w280) -> (x = y?=w286:cluster{"Left":bool, "Top":bool})
        n202 = Unbundle By Name(w286) -> ("Left"=w283:bool)
        n203 = case shown="True" w283 {
          frame False {
            n204 = property on="TRAIN" class="Bool (strict)"("Visible"=TRUE) -> ()  [unwired: 2 in, 2 out]
          }
          frame True {
            w301 = 2 items=["NotSet", "Male", "Female", "Neutral"] ("gender")
            n205 = property on="Yeshwantpur" class="Bool (strict)"("Blinking"=TRUE) -> (error out=w295:errorcluster)  [unwired: 2 in, 1 out]
            n206 = property on="TRAIN" class="Bool (strict)"(error in=w295, "Visible"=FALSE) -> (error out=w296:errorcluster)  [unwired: 1 in, 1 out]
            n207 = constructor class="SpeechSynthesizer"(error in=w296) -> (reference out=w299:refnum<k24>, error out=w300:errorcluster)  [unwired: 2 in, 1 out]
            n208 = invoke class="SpeechSynthesizer" method="SelectVoiceByHints"(reference=w299, error in=w300, "gender"=w301) -> (reference out=w298:refnum<k24>, error out=w302:errorcluster)  [unwired: 1 in, 2 out]
            n209 = invoke class="SpeechSynthesizer" method="Speak"(reference=w298, error in=w302, "textToSpeak"="This stop is Yeshwantpur. The next stop is Nadaprabhu Kempegowda Station, Majestic.") -> ()  [unwired: 1 in, 4 out]
          }
        }
        n210 = Select(t=Control_2."Return to Nadaprabhu Kempegowda Station, Majestic", s=w283, f=Control_2."Return to Yeshwantpur") -> (s? t:f=w284:T1)
        n211 = Decrement(x=w293) -> (x-1=w291:i32)
        n212 = Bundle(w291, "Top"=w292) -> (w287:cluster{i32, "Top":i32})  [unwired: 1 in]
        n213 = property on="TRAIN" class="Bool (strict)"("Position"=w287) -> ()  [unwired: 2 in, 2 out]
      }
      frame "Return to Nadaprabhu Kempegowda Station, Majestic" {
        n214 = Unbundle By Name(w315) -> ("Left"=w318:i32, "Top"=w317:i32)
        n215 = property on="Nadaprabhu\nKemepowda, Majestic" class="Bool (strict)"() -> ("Position"=w305:T2)  [unwired: 2 in, 2 out]
        n216 = property on="Yeshwantpur" class="Bool (strict)"("Blinking"=FALSE) -> ()  [unwired: 2 in, 2 out]
        n217 = property on="TRAIN" class="Bool (strict)"("Visible"=TRUE) -> ()  [unwired: 2 in, 2 out]
        n218 = property on="TRAIN" class="Bool (strict)"() -> ("Position"=w310:T2)  [unwired: 2 in, 2 out]
        n219 = Equal?(x=w310, y=w305) -> (x = y?=w311:cluster{"Left":bool, "Top":bool})
        n220 = Unbundle By Name(w311) -> ("Left"=w308:bool)
        n221 = case shown="True" w308 {
          frame False {
            n222 = property on="TRAIN" class="Bool (strict)"("Visible"=TRUE) -> ()  [unwired: 2 in, 2 out]
          }
          frame True {
            w326 = 2 items=["NotSet", "Male", "Female", "Neutral"] ("gender")
            n223 = property on="TRAIN" class="Bool (strict)"("Visible"=FALSE) -> (error out=w320:errorcluster)  [unwired: 2 in, 1 out]
            n224 = property on="Nadaprabhu\nKemepowda, Majestic" class="Bool (strict)"(error in=w320, "Blinking"=TRUE) -> (error out=w321:errorcluster)  [unwired: 1 in, 1 out]
            n225 = constructor class="SpeechSynthesizer"(error in=w321) -> (reference out=w324:refnum<k24>, error out=w325:errorcluster)  [unwired: 2 in, 1 out]
            n226 = invoke class="SpeechSynthesizer" method="SelectVoiceByHints"(reference=w324, error in=w325, "gender"=w326) -> (reference out=w323:refnum<k24>, error out=w327:errorcluster)  [unwired: 1 in, 2 out]
            n227 = invoke class="SpeechSynthesizer" method="Speak"(reference=w323, error in=w327, "textToSpeak"="This stop is Nadaprabhu Kempegowda Station, Majestic. The next stop is National College.") -> ()  [unwired: 1 in, 4 out]
          }
        }
        n228 = Select(t=Control_2."Return to National College", s=w308, f=Control_2."Return to Nadaprabhu Kempegowda Station, Majestic") -> (s? t:f=w309:T1)
        n229 = Decrement(x=w318) -> (x-1=w316:i32)
        n230 = Bundle(w316, "Top"=w317) -> (w312:cluster{i32, "Top":i32})  [unwired: 1 in]
        n231 = property on="TRAIN" class="Bool (strict)"("Position"=w312) -> ()  [unwired: 2 in, 2 out]
      }
      frame "Return to National College" {
        n232 = Unbundle By Name(w340) -> ("Left"=w343:i32, "Top"=w342:i32)
        n233 = property on="Nadaprabhu\nKemepowda, Majestic" class="Bool (strict)"("Blinking"=FALSE) -> ()  [unwired: 2 in, 2 out]
        n234 = property on="TRAIN" class="Bool (strict)"("Visible"=TRUE) -> ()  [unwired: 2 in, 2 out]
        n235 = Decrement(x=w343) -> (x-1=w341:i32)
        n236 = property on="TRAIN" class="Bool (strict)"() -> ("Position"=w335:T2)  [unwired: 2 in, 2 out]
        n237 = property on="National \nCollege" class="Bool (strict)"() -> ("Position"=w330:T2)  [unwired: 2 in, 2 out]
        n238 = Equal?(x=w335, y=w330) -> (x = y?=w336:cluster{"Left":bool, "Top":bool})
        n239 = Unbundle By Name(w336) -> ("Left"=w333:bool)
        n240 = case shown="True" w333 {
          frame False {
            n241 = property on="TRAIN" class="Bool (strict)"("Visible"=TRUE) -> ()  [unwired: 2 in, 2 out]
          }
          frame True {
            w351 = 2 items=["NotSet", "Male", "Female", "Neutral"] ("gender")
            n242 = property on="TRAIN" class="Bool (strict)"("Visible"=FALSE) -> (error out=w345:errorcluster)  [unwired: 2 in, 1 out]
            n243 = property on="National \nCollege" class="Bool (strict)"(error in=w345, "Blinking"=TRUE) -> (error out=w346:errorcluster)  [unwired: 1 in, 1 out]
            n244 = constructor class="SpeechSynthesizer"(error in=w346) -> (reference out=w349:refnum<k24>, error out=w350:errorcluster)  [unwired: 2 in, 1 out]
            n245 = invoke class="SpeechSynthesizer" method="SelectVoiceByHints"(reference=w349, error in=w350, "gender"=w351) -> (reference out=w348:refnum<k24>, error out=w352:errorcluster)  [unwired: 1 in, 2 out]
            n246 = invoke class="SpeechSynthesizer" method="Speak"(reference=w348, error in=w352, "textToSpeak"="This stop is National College. The next stop is Jayanagar.") -> ()  [unwired: 1 in, 4 out]
          }
        }
        n247 = Select(t=Control_2."Return to Jayanagar", s=w333, f=Control_2."Return to National College") -> (s? t:f=w334:T1)
        n248 = Bundle(w341, "Top"=w342) -> (w337:cluster{i32, "Top":i32})  [unwired: 1 in]
        n249 = property on="TRAIN" class="Bool (strict)"("Position"=w337) -> ()  [unwired: 2 in, 2 out]
      }
      frame "Return to Jayanagar" {
        n250 = Unbundle By Name(w365) -> ("Left"=w368:i32, "Top"=w367:i32)
        n251 = property on="TRAIN" class="Bool (strict)"("Visible"=TRUE) -> ()  [unwired: 2 in, 2 out]
        n252 = property on="National \nCollege" class="Bool (strict)"("Blinking"=FALSE) -> ()  [unwired: 2 in, 2 out]
        n253 = Decrement(x=w368) -> (x-1=w366:i32)
        n254 = property on="Jayanagar" class="Bool (strict)"() -> ("Position"=w355:T2)  [unwired: 2 in, 2 out]
        n255 = property on="TRAIN" class="Bool (strict)"() -> ("Position"=w360:T2)  [unwired: 2 in, 2 out]
        n256 = Equal?(x=w360, y=w355) -> (x = y?=w361:cluster{"Left":bool, "Top":bool})
        n257 = Unbundle By Name(w361) -> ("Left"=w358:bool)
        n258 = case shown="True" w358 {
          frame False {
            n259 = property on="TRAIN" class="Bool (strict)"("Visible"=TRUE) -> ()  [unwired: 2 in, 2 out]
          }
          frame True {
            w376 = 2 items=["NotSet", "Male", "Female", "Neutral"] ("gender")
            n260 = property on="TRAIN" class="Bool (strict)"("Visible"=FALSE) -> (error out=w370:errorcluster)  [unwired: 2 in, 1 out]
            n261 = property on="Jayanagar" class="Bool (strict)"(error in=w370, "Blinking"=TRUE) -> (error out=w371:errorcluster)  [unwired: 1 in, 1 out]
            n262 = constructor class="SpeechSynthesizer"(error in=w371) -> (reference out=w374:refnum<k24>, error out=w375:errorcluster)  [unwired: 2 in, 1 out]
            n263 = invoke class="SpeechSynthesizer" method="SelectVoiceByHints"(reference=w374, error in=w375, "gender"=w376) -> (reference out=w373:refnum<k24>, error out=w377:errorcluster)  [unwired: 1 in, 2 out]
            n264 = invoke class="SpeechSynthesizer" method="Speak"(reference=w373, error in=w377, "textToSpeak"="This stop is Jayanagar. The next stop is Rashtriya Vidyalaya Road.") -> ()  [unwired: 1 in, 4 out]
          }
        }
        n265 = Select(t=Control_2."Return to Rashtriya Vidyalaya Road", s=w358, f=Control_2."Return to Jayanagar") -> (s? t:f=w359:T1)
        n266 = Bundle(w366, "Top"=w367) -> (w362:cluster{i32, "Top":i32})  [unwired: 1 in]
        n267 = property on="TRAIN" class="Bool (strict)"("Position"=w362) -> ()  [unwired: 2 in, 2 out]
      }
      frame "Return to Rashtriya Vidyalaya Road" {
        n268 = Unbundle By Name(w390) -> ("Left"=w393:i32, "Top"=w392:i32)
        n269 = property on="TRAIN" class="Bool (strict)"("Visible"=TRUE) -> ()  [unwired: 2 in, 2 out]
        n270 = property on="Jayanagar" class="Bool (strict)"("Blinking"=FALSE) -> ()  [unwired: 2 in, 2 out]
        n271 = property on="Rashtriya Vidyalaya Road" class="Bool (strict)"() -> ("Position"=w380:T2)  [unwired: 2 in, 2 out]
        n272 = property on="TRAIN" class="Bool (strict)"() -> ("Position"=w385:T2)  [unwired: 2 in, 2 out]
        n273 = Equal?(x=w385, y=w380) -> (x = y?=w386:cluster{"Left":bool, "Top":bool})
        n274 = Unbundle By Name(w386) -> ("Left"=w383:bool)
        n275 = case shown="True" w383 {
          frame False {
            n276 = property on="TRAIN" class="Bool (strict)"("Visible"=TRUE) -> ()  [unwired: 2 in, 2 out]
          }
          frame True {
            w401 = 2 items=["NotSet", "Male", "Female", "Neutral"] ("gender")
            n277 = property on="Rashtriya Vidyalaya Road" class="Bool (strict)"("Blinking"=TRUE) -> (error out=w395:errorcluster)  [unwired: 2 in, 1 out]
            n278 = property on="TRAIN" class="Bool (strict)"(error in=w395, "Visible"=FALSE) -> (error out=w396:errorcluster)  [unwired: 1 in, 1 out]
            n279 = constructor class="SpeechSynthesizer"(error in=w396) -> (reference out=w399:refnum<k24>, error out=w400:errorcluster)  [unwired: 2 in, 1 out]
            n280 = invoke class="SpeechSynthesizer" method="SelectVoiceByHints"(reference=w399, error in=w400, "gender"=w401) -> (reference out=w398:refnum<k24>, error out=w402:errorcluster)  [unwired: 1 in, 2 out]
            n281 = invoke class="SpeechSynthesizer" method="Speak"(reference=w398, error in=w402, "textToSpeak"="This stop is Rashtriya Vidyalaya Road. The next stop is Banashankari .") -> ()  [unwired: 1 in, 4 out]
          }
        }
        n282 = Select(t=Control_2."Return to Banashankari", s=w383, f=Control_2."Return to Rashtriya Vidyalaya Road") -> (s? t:f=w384:T1)
        n283 = Decrement(x=w393) -> (x-1=w391:i32)
        n284 = Bundle(w391, "Top"=w392) -> (w387:cluster{i32, "Top":i32})  [unwired: 1 in]
        n285 = property on="TRAIN" class="Bool (strict)"("Position"=w387) -> ()  [unwired: 2 in, 2 out]
      }
      frame "Return to Banashankari" {
        n286 = Unbundle By Name(w415) -> ("Left"=w418:i32, "Top"=w417:i32)
        n287 = property on="TRAIN" class="Bool (strict)"("Visible"=TRUE) -> ()  [unwired: 2 in, 2 out]
        n288 = property on="Rashtriya Vidyalaya Road" class="Bool (strict)"("Blinking"=FALSE) -> ()  [unwired: 2 in, 2 out]
        n289 = property on="Banashankari" class="Bool (strict)"() -> ("Position"=w405:T2)  [unwired: 2 in, 2 out]
        n290 = property on="TRAIN" class="Bool (strict)"() -> ("Position"=w410:T2)  [unwired: 2 in, 2 out]
        n291 = Equal?(x=w410, y=w405) -> (x = y?=w411:cluster{"Left":bool, "Top":bool})
        n292 = Unbundle By Name(w411) -> ("Left"=w408:bool)
        n293 = case shown="True" w408 {
          frame False {
            n294 = property on="TRAIN" class="Bool (strict)"("Visible"=TRUE) -> ()  [unwired: 2 in, 2 out]
          }
          frame True {
            w426 = 2 items=["NotSet", "Male", "Female", "Neutral"] ("gender")
            n295 = property on="Banashankari" class="Bool (strict)"("Blinking"=TRUE) -> (error out=w420:errorcluster)  [unwired: 2 in, 1 out]
            n296 = property on="TRAIN" class="Bool (strict)"(error in=w420, "Visible"=FALSE) -> (error out=w421:errorcluster)  [unwired: 1 in, 1 out]
            n297 = constructor class="SpeechSynthesizer"(error in=w421) -> (reference out=w424:refnum<k24>, error out=w425:errorcluster)  [unwired: 2 in, 1 out]
            n298 = invoke class="SpeechSynthesizer" method="SelectVoiceByHints"(reference=w424, error in=w425, "gender"=w426) -> (reference out=w423:refnum<k24>, error out=w427:errorcluster)  [unwired: 1 in, 2 out]
            n299 = invoke class="SpeechSynthesizer" method="Speak"(reference=w423, error in=w427, "textToSpeak"="This stop is Banashankari. The next stop is Jaya Prakash Nagar.") -> ()  [unwired: 1 in, 4 out]
          }
        }
        n300 = Select(t=Control_2."Return to Jaya Prakash Nagar", s=w408, f=Control_2."Return to Banashankari") -> (s? t:f=w409:T1)
        n301 = Decrement(x=w418) -> (x-1=w416:i32)
        n302 = Bundle(w416, "Top"=w417) -> (w412:cluster{i32, "Top":i32})  [unwired: 1 in]
        n303 = property on="TRAIN" class="Bool (strict)"("Position"=w412) -> ()  [unwired: 2 in, 2 out]
      }
      frame "Return to Jaya Prakash Nagar" {
        n304 = Unbundle By Name(w440) -> ("Left"=w443:i32, "Top"=w442:i32)
        n305 = property on="Banashankari" class="Bool (strict)"("Blinking"=FALSE) -> ()  [unwired: 2 in, 2 out]
        n306 = property on="TRAIN" class="Bool (strict)"("Visible"=TRUE) -> ()  [unwired: 2 in, 2 out]
        n307 = property on="Jaya Prakash Nagar" class="Bool (strict)"() -> ("Position"=w430:T2)  [unwired: 2 in, 2 out]
        n308 = property on="TRAIN" class="Bool (strict)"() -> ("Position"=w435:T2)  [unwired: 2 in, 2 out]
        n309 = Equal?(x=w435, y=w430) -> (x = y?=w436:cluster{"Left":bool, "Top":bool})
        n310 = Unbundle By Name(w436) -> ("Left"=w433:bool)
        n311 = case shown="True" w433 {
          frame False {
            n312 = property on="TRAIN" class="Bool (strict)"("Visible"=TRUE) -> ()  [unwired: 2 in, 2 out]
          }
          frame True {
            w451 = 2 items=["NotSet", "Male", "Female", "Neutral"] ("gender")
            n313 = property on="TRAIN" class="Bool (strict)"("Visible"=FALSE) -> (error out=w445:errorcluster)  [unwired: 2 in, 1 out]
            n314 = property on="Jaya Prakash Nagar" class="Bool (strict)"(error in=w445, "Blinking"=TRUE) -> (error out=w446:errorcluster)  [unwired: 1 in, 1 out]
            n315 = constructor class="SpeechSynthesizer"(error in=w446) -> (reference out=w449:refnum<k24>, error out=w450:errorcluster)  [unwired: 2 in, 1 out]
            n316 = invoke class="SpeechSynthesizer" method="SelectVoiceByHints"(reference=w449, error in=w450, "gender"=w451) -> (reference out=w448:refnum<k24>, error out=w452:errorcluster)  [unwired: 1 in, 2 out]
            n317 = invoke class="SpeechSynthesizer" method="Speak"(reference=w448, error in=w452, "textToSpeak"="This stop is Jaya Prakash Nagar. The next stop is Yelachenahalli.") -> ()  [unwired: 1 in, 4 out]
          }
        }
        n318 = Select(t=Control_2."Return to Yelachenahalli ", s=w433, f=Control_2."Return to Jaya Prakash Nagar") -> (s? t:f=w434:T1)
        n319 = Decrement(x=w443) -> (x-1=w441:i32)
        n320 = Bundle(w441, "Top"=w442) -> (w437:cluster{i32, "Top":i32})  [unwired: 1 in]
        n321 = property on="TRAIN" class="Bool (strict)"("Position"=w437) -> ()  [unwired: 2 in, 2 out]
      }
      frame "Return to Yelachenahalli " {
        n322 = Unbundle By Name(w465) -> ("Left"=w468:i32, "Top"=w467:i32)
        n323 = property on="Jaya Prakash Nagar" class="Bool (strict)"("Blinking"=FALSE) -> ()  [unwired: 2 in, 2 out]
        n324 = property on="TRAIN" class="Bool (strict)"("Visible"=TRUE) -> ()  [unwired: 2 in, 2 out]
        n325 = Decrement(x=w468) -> (x-1=w466:i32)
        n326 = property on="Yelachenahalli" class="Bool (strict)"() -> ("Position"=w456:T2)  [unwired: 2 in, 2 out]
        n327 = property on="TRAIN" class="Bool (strict)"() -> ("Position"=w460:T2)  [unwired: 2 in, 2 out]
        n328 = Equal?(x=w460, y=w456) -> (x = y?=w461:cluster{"Left":bool, "Top":bool})
        n329 = Unbundle By Name(w461) -> ("Left"=w458:bool)
        n330 = case shown="True" w458 {
          frame False {
            n331 = property on="TRAIN" class="Bool (strict)"("Visible"=TRUE) -> ()  [unwired: 2 in, 2 out]
          }
          frame True {
            w476 = 2 items=["NotSet", "Male", "Female", "Neutral"] ("gender")
            n332 = property on="TRAIN" class="Bool (strict)"("Visible"=FALSE) -> (error out=w470:errorcluster)  [unwired: 2 in, 1 out]
            n333 = property on="Yelachenahalli" class="Bool (strict)"(error in=w470, "Blinking"=TRUE) -> (error out=w471:errorcluster)  [unwired: 1 in, 1 out]
            n334 = constructor class="SpeechSynthesizer"(error in=w471) -> (reference out=w474:refnum<k24>, error out=w475:errorcluster)  [unwired: 2 in, 1 out]
            n335 = invoke class="SpeechSynthesizer" method="SelectVoiceByHints"(reference=w474, error in=w475, "gender"=w476) -> (reference out=w473:refnum<k24>, error out=w477:errorcluster)  [unwired: 1 in, 2 out]
            n336 = invoke class="SpeechSynthesizer" method="Speak"(reference=w473, error in=w477, "textToSpeak"="This stop is Yelachenahalli. This is the last stop. ") -> ()  [unwired: 1 in, 4 out]
          }
        }
        n337 = Select(t=Control_2."Stop", s=w458, f=Control_2."Return to Yelachenahalli ") -> (s? t:f=w459:T1)
        n338 = Bundle(w466, "Top"=w467) -> (w462:cluster{i32, "Top":i32})  [unwired: 1 in]
        n339 = property on="TRAIN" class="Bool (strict)"("Position"=w462) -> ()  [unwired: 2 in, 2 out]
      }
      frame "Stop" {
        n340 = property on="TRAIN" class="Bool (strict)"() -> ("Position"=w485:T2)  [unwired: 2 in, 2 out]
        n341 = Equal?(x=w484, y=w485) -> (x = y?=w483:cluster{"Left":bool, "Top":bool})
        n342 = Unbundle By Name(w483) -> ("Left"=w482:bool, "Top"=w481:bool)
        n343 = And(x=w482, y=w481) -> (x .and. y?=w480:bool)
      }
    }
    n344 = Or(x="Stop", y=w4) -> (x .or. y?=w3:bool)
    n345 = case shown="True" "Stop" {
      frame False {
      }
      frame True {
        n346 = property on="TRAIN" class="Bool (strict)"("Visible"=TRUE) -> ()  [unwired: 2 in, 2 out]
        n347 = property on="TRAIN" class="Bool (strict)"("Position"=T2 {"Left"=478, "Top"=442}) -> ()  [unwired: 2 in, 2 out]
      }
    }
  }
